vi "ReportADCResultsInVoltsTSFTS2_v2.vi"(6 "Blue Board Enum":T1=enum."INVB_UDC", 7 "Green Board Enum":T3, 8 "error in (no error)":errorcluster, 9 "Message IN":string, 10 "Board Selector":T2, 11 "Control Board VISA":refnum<visa-resource-name>) -> (0 "error out":errorcluster, 1 "Message OUT":string, 2 "Result":dbl, 3 "Control Board VISA Out":refnum<visa-resource-name>)   [LabVIEW 2022 SP3]
uses:
  ADCSelector GB.ctl
  Board Select.ctl
  ADCSelector BB.ctl
  <vilib>/Instr/_visa.llb/VISA Flush IO Buffer Mask.ctl
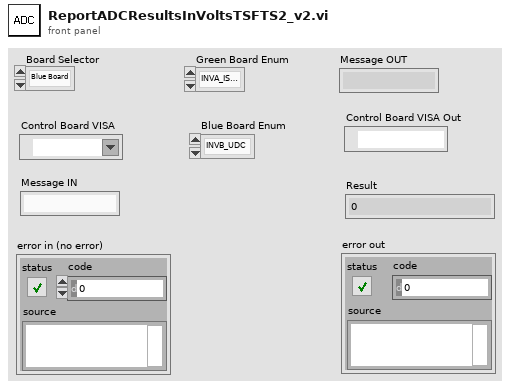
[diagram p1: front panel]
types:
  T1 = typedef "ADCSelector BB.ctl" = enum16{"INVA_ISENSE_U", "INVA_ISENSE_V", "INVA_ISENSE_W", "INVA_UDC", "INVA_TEMP", "HB_TEMP", "AUXB_TEMP", "VLINE_AB", "VLINE_BC", "VLINE_CA", "VSENSE_POS_24V", "VSENSE_POS_5V", "VSENSE_NEG_15V", "INVB_ISENSE_U", "INV_B_ISENSEV", "INVB_ISENSE_W", "INVB_UDC", "INVB_TEMP", "AUXA_TEMP", "AUXC_TEMP", "VOUT_AB", "VOUT_BC", "VOUT_CA", "VSENSE_POS_15V", "VSENSE_POS_3P3V", "TEST_POINT"}
  T2 = typedef "Board Select.ctl" = enum16{"Blue Board", "Green Board"}
  T3 = typedef "ADCSelector GB.ctl" = enum16{"INVA_ISENSE_U", "INVA_ISENSE_V", "INVA_ISENSE_W", "INVA_UDC", "INVA_TEMP", "HB_ISENSE", "AUX_ISENSE_U", "AUX_ISENSE_V", "AUX_ISENSE_W", "VLINE_AB", "VLINE_BC", "VLINE_CA", "REF_1P5V", "VSENSE_POS_24V", "VSENSE_POS_5V", "VSENSE_NEG_15V", "TEST_POINT", "INVB_ISENSE_U", "INVB_ISENSE_V", "INVB_ISENSE_W", "INVB_UDC", "INVB_TEMP", "HB_TEMP", "AUXA_TEMP", "AUXB_TEMP", "AUXC_TEMP", "VOUT_AB", "VOUT_BC", "VOUT_CA", "REF_2P5V", "VSENSE_POS_15V", "VSENSE_POS_3P3V", "NET_ANALYZER"}
  T4 = typedef "VISA Flush IO Buffer Mask.ctl" = u16
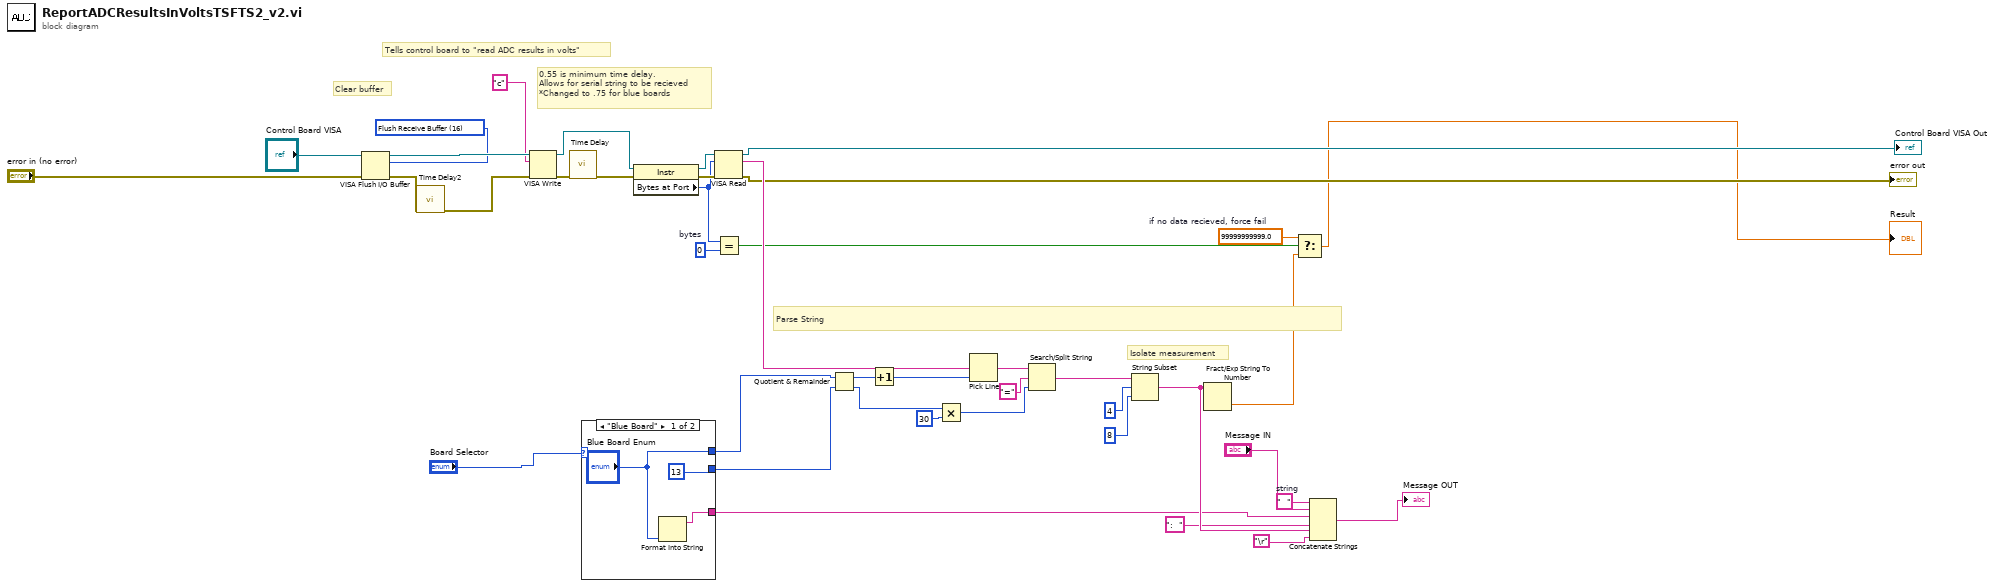
[diagram p0: block diagram]
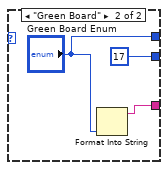
[diagram p2: hidden frame]
diagram:
  w12 = "  "  # string
  w18 = 99999999999.0  # if no data recieved, force fail
  w21 = u32 0  # bytes
  w26 = T4 16 items=["Flush Receive Buffer"=16, "Write Transmit Buffer to Device"=32, "Flush Receive Buffer (No I/O)"=64, "Flush Transmit Buffer"=128] ("Mask")
  # "Isolate measurement"
  # "Clear buffer"
  # "Parse String"
  # "0.55 is minimum time delay.\nAllows for serial string to be recieved\n*Changed to .75 for blue boards"
  # "Tells control board to \"read ADC results in volts\""
  n1 = VISA Flush I/O Buffer(VISA resource name="Control Board VISA", mask (16)=w26, error in (no error)="error in (no error)") -> (VISA resource name out=w28:refnum<visa-resource-name>, error out=w3:errorcluster)
  n2 = call "Time Delay2"("error in (no error)"=w3) -> ("error out"=w2:errorcluster)  [unwired: 10 in]
  n3 = VISA Write(VISA resource name=w28, write buffer="c", error in (no error)=w2) -> (VISA resource name out=w30:refnum<visa-resource-name>, error out=w27:errorcluster)  [unwired: 1 out]
  n4 = call "Time Delay"("error in (no error)"=w27) -> ("error out"=w29:errorcluster)  [unwired: 10 in]
  n5 = case shown="\"Blue Board\"" "Board Selector" {
    tunnel: ["Blue Board Enum" "Green Board Enum"] -> w7
    tunnel: [13 17] -> w6
    tunnel: [w43 w45] -> w5
    frame "Blue Board" {
      n6 = Format Into String("Blue Board Enum") -> (resulting string=w43:string)  [unwired: 3 in, 1 out]
    }
    frame "Green Board" {
      n7 = Format Into String("Green Board Enum") -> (resulting string=w45:string)  [unwired: 3 in, 1 out]
    }
  }
  n8 = property class="Instr"(reference=w30, error in=w29) -> (reference out=w24:refnum<visa-resource-name>, error out=w25:errorcluster, "Bytes at Port"=w22:u32)
  n9 = VISA Read(VISA resource name=w24, byte count=w22, error in (no error)=w25) -> (VISA resource name out=→"Control Board VISA Out":refnum<visa-resource-name>, read buffer=w39:string, error out=→"error out":errorcluster)  [unwired: 1 out]
  n10 = Equal?(x=w22, y=w21) -> (x = y?=w19:bool)
  n11 = Quotient & Remainder(x=w7, y=w6) -> (x-y*floor(x/y)=w34:i32, floor(x/y)=w36:i32)
  n12 = Increment(x=w34) -> (x+1=w35:i32)
  n13 = Multiply(x=w36, y=30) -> (x*y=w38:i32)
  n14 = Pick Line(multi-line string=w39, line index=w35) -> (output string=w40:string)  [unwired: 1 in]
  n15 = Search/Split String(string=w40, search string/char (-)="=" ("regular expression"), offset (0)=w38) -> (match + rest of string=w32:string)  [unwired: 2 out]
  n16 = String Subset(string=w32, offset (0)=4, length (rest)=8 ("offset (0)")) -> (substring=w14:string)
  n17 = Fract/Exp String To Number(string=w14) -> (number=w20:dbl)  [unwired: 3 in, 1 out]
  n18 = Select(t=w18, s=w19, f=w20) -> (s? t:f=→"Result":dbl)
  n19 = Concatenate Strings(w12, "Message IN", w5, ":  ", w14, "\r") -> (→"Message OUT":string)
